vi "sub_make_safe_name.vi"(11 "Input String":string) -> (3 "Safe Output String":string)   [LabVIEW 2013, in "daqio minimal.lvlib"]
doc: "This VI will replace all special characters with \"_\" (underscores) and will only allow numbers and capital letters. This way, the output string can safely be used as a KEY on daq.io."
uses:
  daqio minimal.lvlib
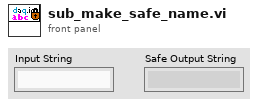
[diagram p1: front panel]
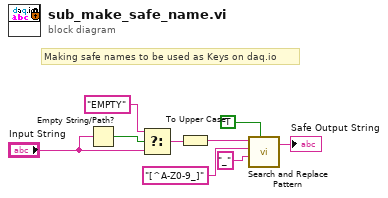
[diagram p0: block diagram]
diagram:
  # "Making safe names to be used as Keys on daq.io"
  n1 = Empty String/Path?(string/path="Input String") -> (empty?=w4:bool)
  n2 = Select(t="EMPTY", s=w4, f="Input String") -> (s? t:f=w1:string)
  n3 = To Upper Case(1:w1) -> (0:w5:string)
  n4 = call <vilib>:"Search and Replace Pattern.vi"("string"=w5, "regular expression (\"\")"="[^A-Z0-9_]" ("regular expression (\"\")"), "replace string (\"\")"="_" ("replace string (\"\")"), "replace all? (F)"=TRUE) -> ("result string"=→"Safe Output String":string)  [unwired: 1 in, 1 out]
